vi "http parse header string.vi"(11 "raw string":string) -> (0 "no field name":bool, 1 "no crlf":bool, 2 "header field data":string, 3 "header field name":string)   [LabVIEW 2013]
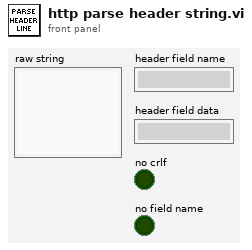
[diagram p1: front panel]
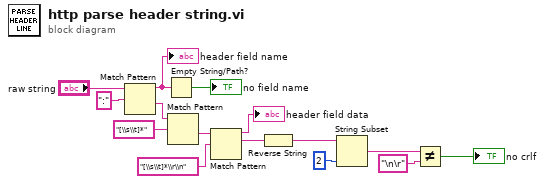
[diagram p0: block diagram]
diagram:
  n1 = Match Pattern(string="raw string", regular expression=":") -> (before substring=w2:string, after substring=w11:string)  [unwired: 1 in, 2 out]
  "header field name" <- w2
  n2 = Empty String/Path?(string/path=w2) -> (empty?=→"no field name":bool)
  n3 = Match Pattern(string=w11, regular expression="[\\s\\t]*") -> (after substring=w13:string)  [unwired: 1 in, 3 out]
  n4 = Match Pattern(string=w13, regular expression="[\\s\\t]*\\r\\n") -> (before substring=→"header field data":string, match substring=w8:string)  [unwired: 1 in, 2 out]
  n5 = Reverse String(1:w8) -> (0:w7:string)
  n6 = String Subset(string=w7, length (rest)=2 ("length (rest)")) -> (substring=w5:string)  [unwired: 1 in]
  n7 = Not Equal?(x=w5, y="\n\r" ("regular expression")) -> (x != y?=→"no crlf":bool)
